vi "EnableDisableGainRing.vi"(8 "error in (no error)":errorcluster, 10 "Bool Refnum":refnum<vi>, 11 "Ring in":refnum<vi>) -> (0 "error out":errorcluster)   [LabVIEW 2016]
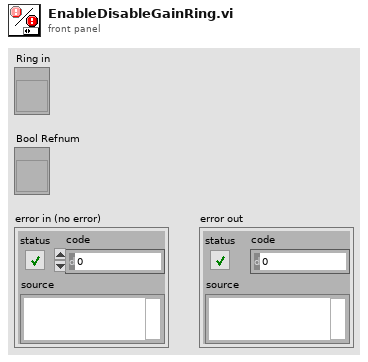
[diagram p1: front panel]
types:
  T1 = enum8{"Enabled", "Disabled", "Disabled and Grayed Out"}
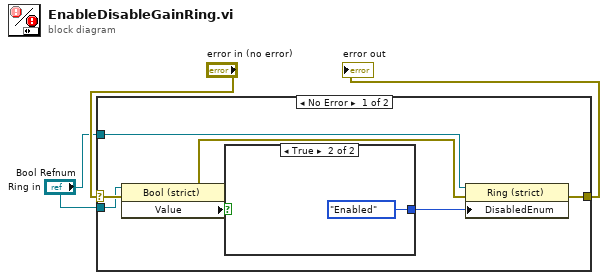
[diagram p0: block diagram]
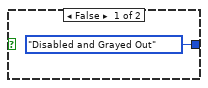
[diagram p2: hidden frame]
diagram:
  n1 = case shown="No Error" "error in (no error)" {
    selector: "error in (no error)" -> [w8 w14]
    tunnel: [w7 w14] -> w4
    tunnel: "Ring in" -> [w6 _]
    tunnel: "Bool Refnum" -> [w5 _]
    frame No Error {
      n2 = property on="Property Node" class="Bool (strict)"(reference=w5, error in=w8) -> (error out=w9:errorcluster, "Value"=w11:bool)  [unwired: 1 out]
      n3 = case shown="True" w11 {
        tunnel: [T1."Disabled and Grayed Out" ("Disabled") T1."Enabled" ("Disabled")] -> w10
        frame False {
        }
        frame True {
        }
      }
      n4 = property on="Property Node" class="Ring (strict)"(reference=w6, error in=w9, "DisabledEnum"=w10) -> (error out=w7:errorcluster)  [unwired: 1 out]
    }
    frame Error {
    }
  }
  "error out" <- w4
